vi "Integrate channel from file.vi"(4 "Buffer size":i64=1048576 format="%d (0x%x)", 5 "Offset correction":dbl, 6 "Offset duration":dbl=0.0095, 7 "group name":string="Untitled", 8 "Error In":errorcluster, 9 "Save data":bool, 10 "Integration settings":T1={"Channel"="CH0", "Output name"="Integral", "Factor"=-137722.0, "Start time"=0.0, "Duration"=3.0, "Fix drift"=FALSE} {"Duration" format="%#_6ps"; "Start time" format="%#_6ps"}, 11 "File Path Control":path=path "\\\\eden\\NHMFLDATA/Data/Generator/December_2015/121715/rp163145_121715.tdms") -> (0 "Error Out":errorcluster, 1 "Integrated Waveform":waveform(dbl), 2 "Min max":cluster{"Max":dbl, "Min":dbl}, 3 "File Path out":path)   [LabVIEW 2016]
uses:
  Utilities/Controls/Integrate channel.ctl
  <vilib>/Waveform/WDTOps.llb/WDT Number of Waveform Samples DBL.vi
  <vilib>/Waveform/WDTOps.llb/WDT Append Waveforms DBL.vi
panel:
  out "Waveform Graph":waveform(dbl)(graph)
  # "Input CH            Factor              Output CH      Start              Duration"
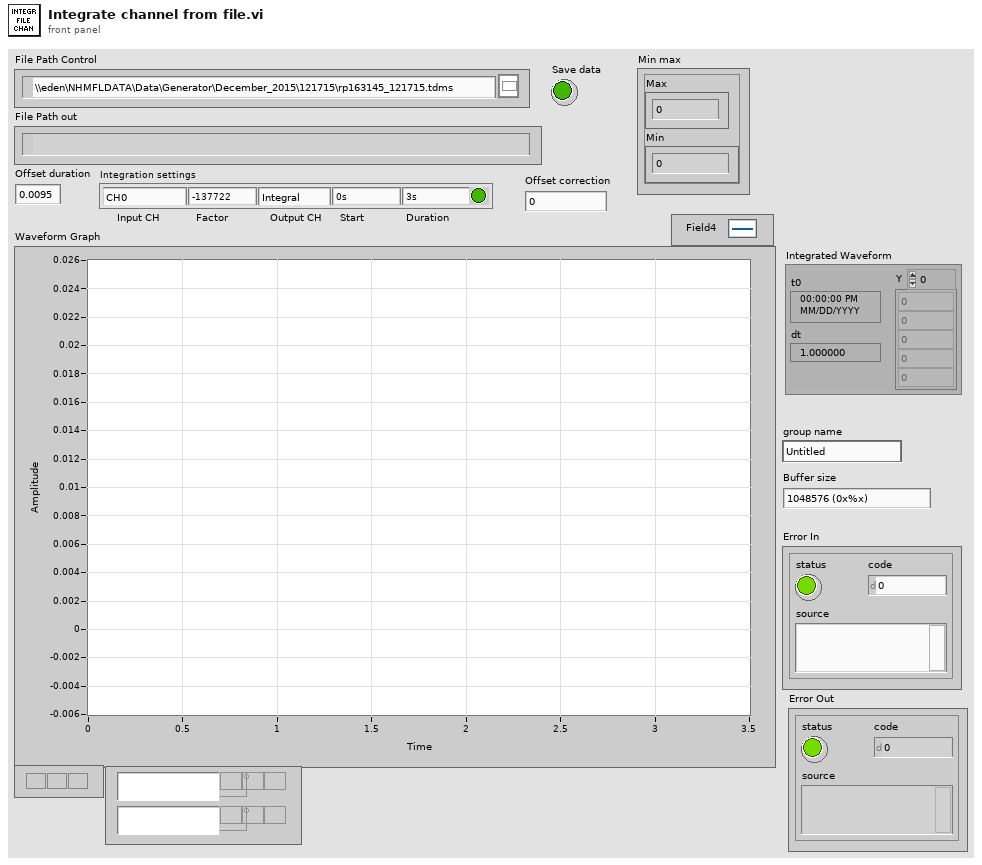
[diagram p1: front panel]
types:
  T1 = typedef "Integrate channel.ctl" = cluster{"Channel":string, "Output name":string, "Factor":dbl, "Start time":dbl, "Duration":dbl, "Fix drift":bool}
  T2 = enum16{"open", "open or create", "create or replace", "create", "open (read-only)"}
  T3 = typedef "TDMS channel info.ctl" = cluster{"t0":timestamp, "dt":dbl, "Channel length":i64}
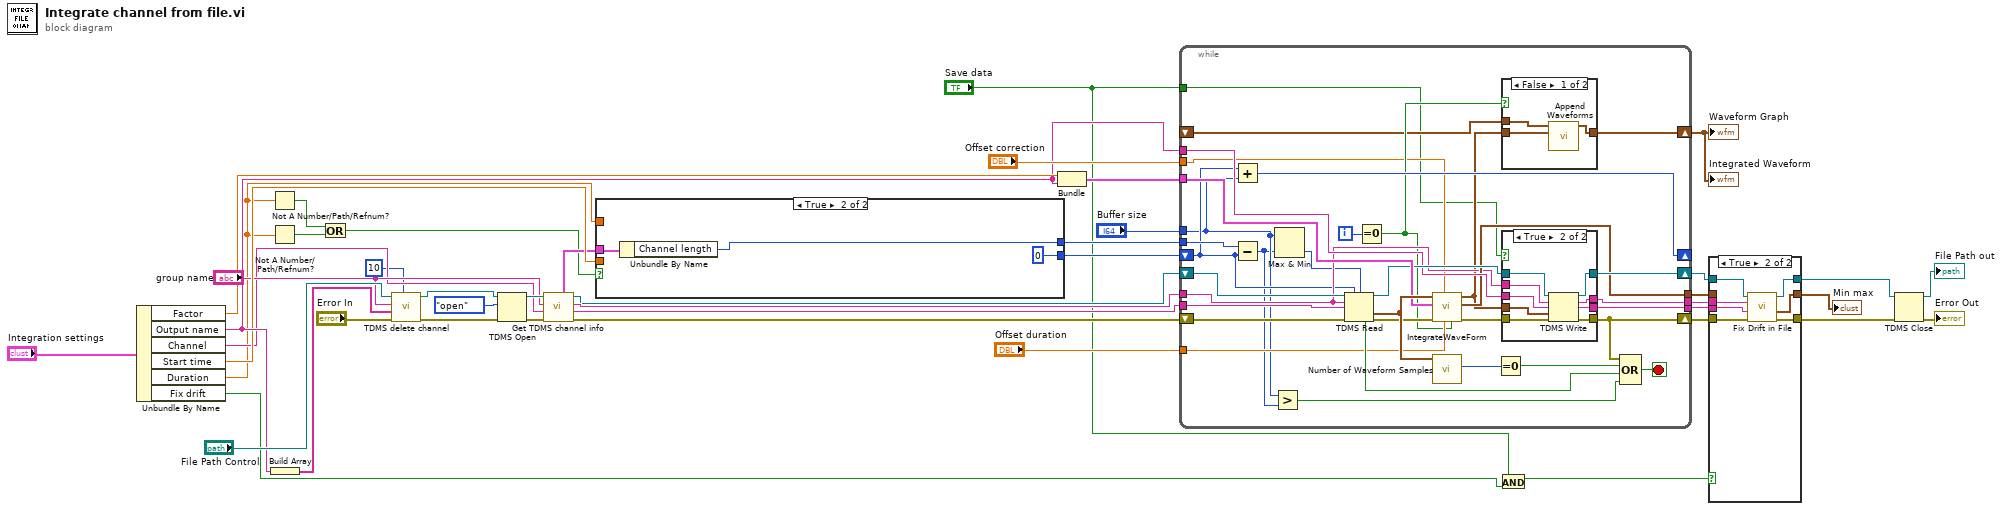
[diagram p0: block diagram]
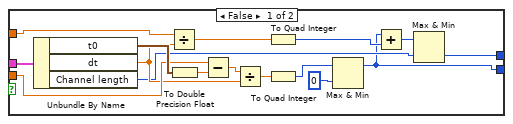
[diagram p3: hidden frame]
diagram:
  n1 = Unbundle By Name("Integration settings") -> ("Factor"=w42:dbl, "Output name"=w31:string, "Channel"=w24:string, "Start time"=w29:dbl, "Duration"=w16:dbl, "Fix drift"=w4:bool)
  n2 = Not A Number/Path/Refnum?(number/path/refnum=w16) -> (NaN/Path/Refnum?=w15:bool)
  n3 = Not A Number/Path/Refnum?(number/path/refnum=w16) -> (NaN/Path/Refnum?=w14:bool)
  n4 = Build Array(w31) -> (w30:string[])
  n5 = Or(x=w15, y=w14) -> (x .or. y?=w13:bool)
  n6 = call "TDMS delete channel.vi"("Delay"=u32 10, "error in (no error)"="Error In", "Channels"=w30, "group name"="group name", "file path"="File Path Control") -> ("error out"=w32:errorcluster, "file path out"=w34:path)  [unwired: 4 in, 1 out]
  n7 = TDMS Open(8:w32, 10:T2."open" ("operation (0:open)"), 11:w34) -> (0:w27:errorcluster, 3:w26:refnum<k34>)  [unwired: 4 in]
  n8 = call "Get TDMS channel info.vi"("error in"=w27, "Channel name"=w24, "group name"="group name", "tdms file"=w26) -> ("error out"=w20:errorcluster, "channel name out"=w22:string, "group name out"=w23:string, "tdms file out"=w21:refnum<k34>, "TDMS channel info"=w19:T3)  [unwired: 3 in]
  n9 = case shown="True" w13 {
    tunnel: w29 -> [w58 _]
    tunnel: w16 -> [w57 _]
    tunnel: [w45 i64 0] -> w28
    tunnel: w19 -> [w53 w62]
    tunnel: [w48 w61] -> w18
    frame False {
      n10 = Unbundle By Name(w53) -> ("t0"=w60:timestamp, "dt"=w56:dbl, "Channel length"=w50:i64)
      n11 = Divide(x=w57, y=w56) -> (x/y=w49:dbl)
      n12 = To Double Precision Float(number=w60) -> (double precision float=w59:dbl)
      n13 = Subtract(x=w58, y=w59) -> (x-y=w52:dbl)
      n14 = Divide(x=w52, y=w56) -> (x/y=w55:dbl)
      n15 = To Quad Integer(1:w49) -> (0:w46:i64)
      n16 = To Quad Integer(1:w55) -> (0:w54:i64)
      n17 = Max & Min(x=w54, y=i64 0) -> (max(x,y)=w45:i64)  [unwired: 1 out]
      n18 = Add(x=w45, y=w46) -> (x+y=w47:i64)
      n19 = Max & Min(x=w47, y=w50) -> (min(x,y)=w48:i64)  [unwired: 1 out]
    }
    frame True {
      n20 = Unbundle By Name(w62) -> ("Channel length"=w61:i64)
    }
  }
  n21 = Bundle("Factor"=w42, "Output name"=w31) -> (w41:cluster{"Factor":dbl, "Output name":string})  [unwired: 1 in]
  n22 = while {
    tunnel: w22 -> [w95]
    tunnel: w41 -> [w93]
    tunnel: w31 -> [w91]
    shift-right: [w84] -> w10
    shift-left: w20 -> [w87]
    shift-right: [w85] -> w12
    shift-left: w21 -> [w97]
    tunnel: "Buffer size" -> [w69]
    shift-right: [w82] -> _
    shift-left: w28 -> [w71]
    tunnel: "Offset duration" -> [w80]
    tunnel: [w79] -> w7
    tunnel: w23 -> [w78]
    shift-right: [w76] -> w17
    shift-left: _ -> [w74]
    tunnel: "Offset correction" -> [w73]
    tunnel: w18 -> [w72]
    tunnel: [w66] -> w6
    tunnel: "Save data" -> [w65]
    tunnel: [w64] -> w2
    i -> [w81]
    stop <- w86 stop-if-true
    n23 = Add(x=w71, y=w69) -> (x+y=w82:i64)
    n24 = Subtract(x=w72, y=w71) -> (x-y=w68:i64)
    n25 = Greater?(x=w69, y=w68) -> (0:w67:bool)
    n26 = Max & Min(x=w69, y=w68) -> (min(x,y)=w70:i64)  [unwired: 1 out]
    n27 = TDMS Read(0:w97, 1:w71, 2:w70, 5:w78, 7:w95, 11:w87) -> (4:w92:refnum<k34>, 10:w94:waveform(dbl), 14:w83:bool, 15:w90:errorcluster)  [unwired: 2 in, 2 out]
    n28 = Equal To 0?(x=w81) -> (x = 0?=w77:bool)
    n29 = call "IntegrateWaveForm.vi"("First chunk?"=w77, "Offset duration"=w80, "Offset correction"=w73, "error in (no error)"=w90, "Integrate settings"=w93, "Waveform"=w94) -> ("error out"=w89:errorcluster, "Min max"=w79:cluster{"Max":dbl, "Min":dbl}, "Integrated Waveform"=w75:waveform(dbl))  [unwired: 3 in]
    n30 = call-poly <vilib>:"Number of Waveform Samples.vi"("waveform in"=w94) -> ("number of samples"=w96:i32)  [unwired: 8 in, 2 out]
    n31 = Equal To 0?(x=w96) -> (x = 0?=w88:bool)
    n32 = case shown="False" w77 {
      tunnel: [w98 w101] -> w76
      tunnel: w75 -> [w99 w101]
      tunnel: w74 -> [w100 _]
      frame False {
        n33 = call-poly <vilib>:"Append Waveforms.vi"("waveform B"=w99, "waveform A"=w100) -> ("waveform out"=w98:waveform(dbl))  [unwired: 8 in, 1 out]
      }
      frame True {
      }
    }
    n34 = case shown="True" w65 {
      tunnel: w92 -> [w105 w114]
      tunnel: w91 -> [w103 w113]
      tunnel: w75 -> [_ w112]
      tunnel: w89 -> [w104 w111]
      tunnel: [w105 w110] -> w85
      tunnel: [w104 w109] -> w84
      tunnel: w78 -> [w102 w108]
      tunnel: [w103 w107] -> w66
      tunnel: [w102 w106] -> w64
      frame False {
      }
      frame True {
        n35 = TDMS Write(0:w114, 5:w108, 7:w113, 9:w112, 11:w111) -> (4:w110:refnum<k34>, 6:w106:string, 8:w107:string, 15:w109:errorcluster)  [unwired: 1 in]
      }
    }
    n36 = Compound Arithmetic op=OR(w84, w88, w83, w67) -> (w86:bool)
  }
  "Integrated Waveform" <- w17
  "Waveform Graph" <- w17
  n37 = And(x="Save data", y=w4) -> (x .and. y?=w5:bool)
  n38 = case shown="True" w5 {
    tunnel: w12 -> [w115 w124]
    tunnel: [w115 w123] -> w11
    tunnel: w10 -> [w116 w122]
    tunnel: [w116 w121] -> w9
    tunnel: [w117 w120] -> w8
    tunnel: w7 -> [w117 _]
    tunnel: w6 -> [_ w119]
    tunnel: w2 -> [_ w118]
    frame False {
    }
    frame True {
      n39 = call "Fix Drift in File.vi"("error in (no error)"=w122, "channel name(s) in"=w119, "group name"=w118, "tdms file"=w124) -> ("error out"=w121:errorcluster, "Min max"=w120:cluster{"Max":dbl, "Min":dbl}, "tdms file out"=w123:refnum<k34>)  [unwired: 3 in, 2 out]
    }
  }
  "Min max" <- w8
  n40 = TDMS Close(8:w9, 11:w11) -> (0:→"Error Out":errorcluster, 3:→"File Path out":path)
